vi "SendSoftwareTrigger.vi"(8 "error in (no error)":errorcluster, 11 "Keysight44xx in":refnum<class "Keysight44xx.lvclass">) -> (0 "error out":errorcluster, 3 "Keysight44xx out":refnum<class "Keysight44xx.lvclass">)   [LabVIEW 2018, in "SpecAnPlugins.lvlib" / "Keysight44xx.lvclass"]
doc: "This function sends a software trigger to the Spectrum Analyzer in order to begin acquisition."
uses:
  Keysight44xx.lvclass
  C:/Users/ico/Documents/Projects/NistPluggableModules/SpecAn/SpecAnPlugins/SpecAnBaseClass/SpecAnBase.lvclass
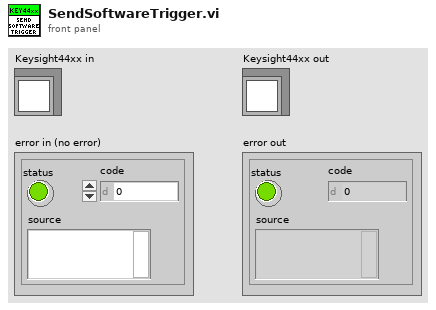
[diagram p1: front panel]
types:
  T1 = typedef "SpecAnPlugins.lvlib/SpecAnBase.lvclass/Acquisition.ctl" = cluster{"Handle":string, "Connected":bool, "Enabled":bool, "SweepModeContinuous":bool, "NumberOfSweeps":i32, "DetectorTypeAuto":bool, "DetectorType":i32, "VerticalScale":i32, "MaximumTime(seconds)":dbl}
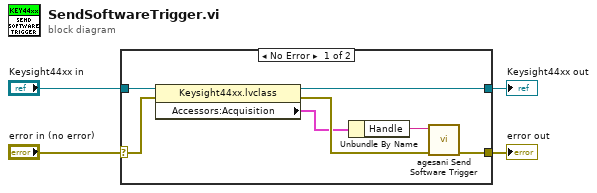
[diagram p0: block diagram]
diagram:
  n1 = case shown="No Error" "error in (no error)" {
    selector: "error in (no error)" -> [w10 w13]
    tunnel: [w8 w13] -> w3
    tunnel: "Keysight44xx in" -> [w11 w12]
    tunnel: [w7 w12] -> w1
    frame No Error {
      n2 = property class="Keysight44xx.lvclass"(reference=w11, error in=w10) -> (reference out=w7:refnum<class "Keysight44xx.lvclass">, error out=w9:errorcluster, "Accessors:Acquisition"=w6:T1)
      n3 = Unbundle By Name(w6) -> ("Handle"=w5:string)
      n4 = call <instrlib>:"agesani Send Software Trigger.vi"("error in (no error)"=w9, "instrument handle"=w5) -> ("error out"=w8:errorcluster)  [unwired: 8 in, 1 out]
    }
    frame Error {
    }
  }
  "error out" <- w3
  "Keysight44xx out" <- w1
